vi "parse_float32.vi"   [LabVIEW 2010]
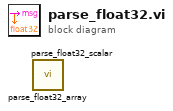
[diagram p0: block diagram]
diagram:
  n1 = call "parse_float32_array.vi"() -> ()  [unwired: 5 in, 3 out]
  n2 = call "parse_float32_scalar.vi"() -> ()  [unwired: 5 in, 3 out]
